vi "20150814 Ultrasonic distance measurements.vi"(0 "Serial Port":refnum<visa-resource-name>="COM10", 1 "Action":enum16{"Initialize", "Close", "Read distance"}(ring), 5 "LINX Resource in":T1, 7 "Trig":u8=48, 9 "Echo Pin (DI)":u8=49, 11 "error in (no error)":errorcluster) -> (4 "Serial Port out":refnum<visa-resource-name>="COM10", 6 "LINX Resource out":T1, 8 "UL sensor initialize OK?":bool, 10 "Distance(cm)":dbl, 15 "Error Out":errorcluster)   [LabVIEW 2013]
uses:
  <vilib>/MakerHub/LINX/Private/Type Defs/LINX Ref.ctl
  <vilib>/MakerHub/LINX/Private/Type Defs/Platform.ctl
  <vilib>/MakerHub/LINX/Private/Type Defs/Interface.ctl
  <vilib>/MakerHub/LINX/Private/Device/Type Defs/LINX Device Config.ctl
  <vilib>/MakerHub/LINX/Private/Device/Type Defs/TCP Config.ctl
  <vilib>/MakerHub/LINX/Private/Device/Type Defs/Channels.ctl
  <vilib>/MakerHub/LINX/LMH-LINX.lvlib
  <vilib>/MakerHub/LINX/Public/Sensors/Ultrasonic/Ultrasonic.lvlib
  <vilib>/MakerHub/LINX/Private/Device/Device.lvlib
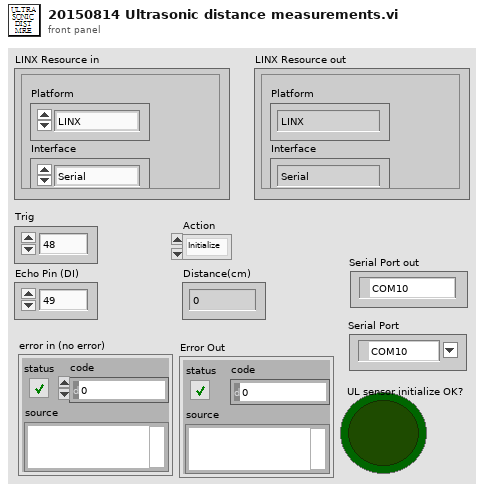
[diagram p1: front panel]
types:
  T1 = typedef "LMH-LINX.lvlib/LINX Ref.ctl" = cluster{"Platform":T2, "Interface":T3, "LINX Device Config":T4}
  T2 = typedef "LMH-LINX.lvlib/Platform.ctl" = enum16{"LINX", "myRIO"}
  T3 = typedef "LMH-LINX.lvlib/Interface.ctl" = enum16{"Serial", "TCP"}
  T4 = typedef "LMH-LINX.lvlib/Device.lvlib/LINX Device Config.ctl" = cluster{"Interface":T3, "COM Port":refnum<visa-resource-name>, "TCP Configuration":T5, "Device Family":u8, "Device ID":u8, "Device Name":string, "TCP Ref":refnum<k5>, "Channels":T6}
  T5 = typedef "LMH-LINX.lvlib/Device.lvlib/TCP Config.ctl" = cluster{"IP Address":string, "Port":u16}
  T6 = typedef "LMH-LINX.lvlib/Channels.ctl" = cluster{"DI":u8[], "DO":u8[], "AI":u8[], "AO":u8[], "PWM":u8[], "QE":u8[], "UART":u8[], "I2C 2":u8[], "SPI":u8[], "CAN":u8[], "Servo":u8[], "AI Ref (V)":dbl, "AO Ref (V)":dbl, "AO Resolution (Bits)":u8}
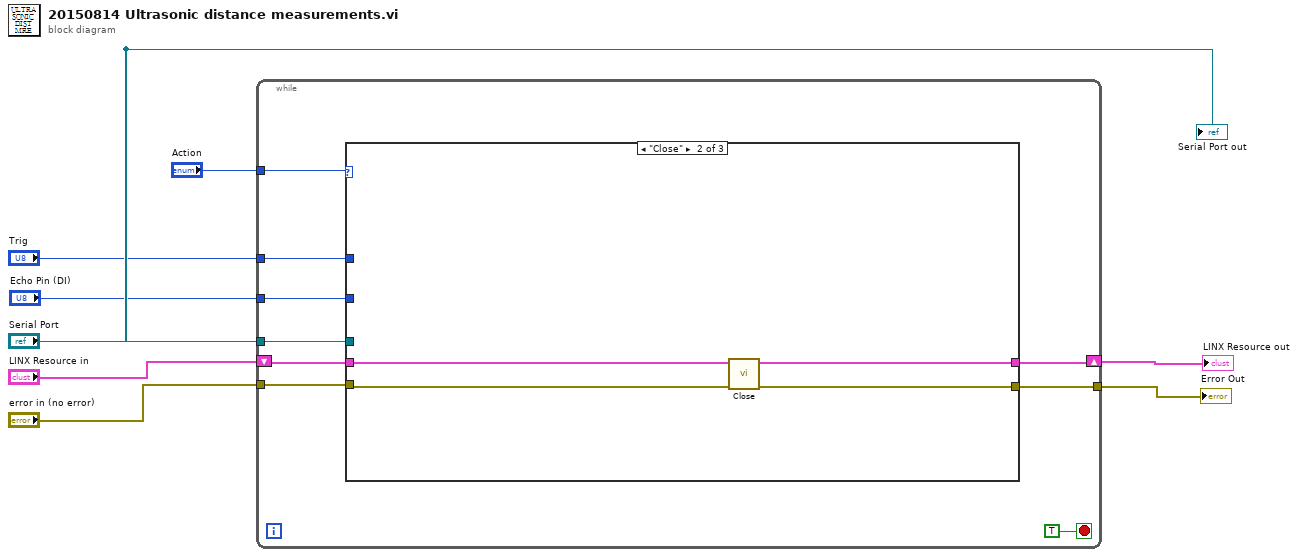
[diagram p0: block diagram]
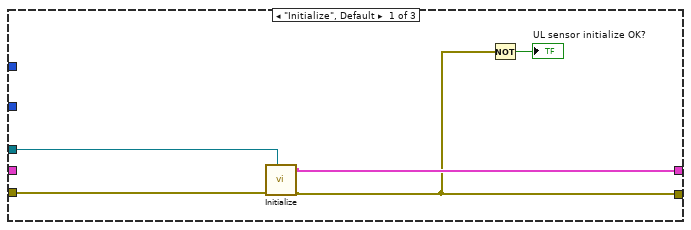
[diagram p2: hidden frame]
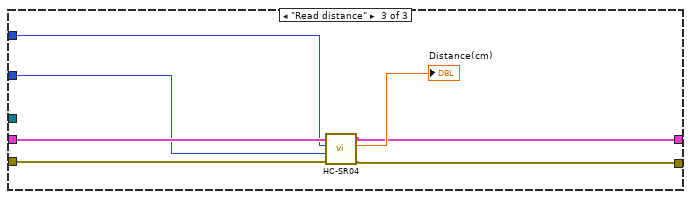
[diagram p3: hidden frame]
diagram:
  n1 = while {
    tunnel: "Action" -> [w17]
    tunnel: "error in (no error)" -> [w15]
    tunnel: [w14] -> w7
    tunnel: "Serial Port" -> [w13]
    shift-right: [w12] -> w1
    shift-left: "LINX Resource in" -> [w11]
    tunnel: "Trig" -> [w10]
    tunnel: "Echo Pin (DI)" -> [w9]
    stop <- TRUE stop-if-true
    n2 = case shown="\"Close\"" w17 {
      tunnel: w15 -> [w21 w23 w31]
      tunnel: [w18 w26 w29] -> w14
      tunnel: w13 -> [w20 _ _]
      tunnel: [w19 w25 w30] -> w12
      tunnel: w11 -> [_ w24 w32]
      tunnel: w10 -> [_ _ w28]
      tunnel: w9 -> [_ _ w27]
      frame "Initialize", Default {
        n3 = call <vilib>:"Initialize.vi"("Serial Port"=w20, "Error In"=w21) -> ("Error Out"=w18:errorcluster, "LINX Ref"=w19:T1)  [unwired: 7 in, 1 out]
        n4 = Not(x=w18) -> (.not. x?=→"UL sensor initialize OK?":bool)
      }
      frame "Close" {
        n5 = call <vilib>:"Close.vi"("Error In"=w23, "LINX Resource"=w24) -> ("Error Out"=w26:errorcluster, "LINX Resource"=w25:T1)  [unwired: 8 in]
      }
      frame "Read distance" {
        n6 = call <vilib>:"HC-SR04.vi"("Error In"=w31, "Echo Pin (DI)"=w27, "Trig"=w28, "LINX Resource"=w32) -> ("Error Out"=w29:errorcluster, "Centimeters"=→"Distance(cm)":dbl, "LINX Resource"=w30:T1)  [unwired: 4 in, 1 out]
      }
    }
  }
  "Error Out" <- w7
  "LINX Resource out" <- w1
  "Serial Port out" <- "Serial Port"
